vi "Evaluate Population Fitness.vi"(8 "error in":errorcluster, 11 "IPopulation in":refnum<class "IPopulation.lvclass">) -> (0 "error out":errorcluster, 3 "IPopulation out":refnum<class "IPopulation.lvclass">)   [LabVIEW 2016, in "IPopulation.lvclass"]
uses:
  IPopulation.lvclass
  IPopulation.lvclass/IPopulation.ctl
  IChromosome/IChromosome.lvclass
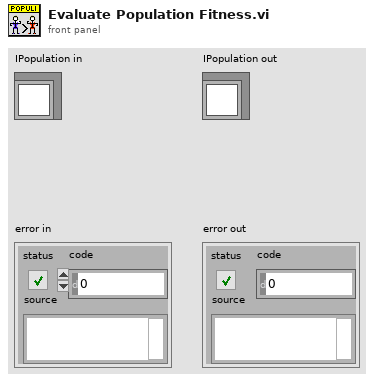
[diagram p1: front panel]
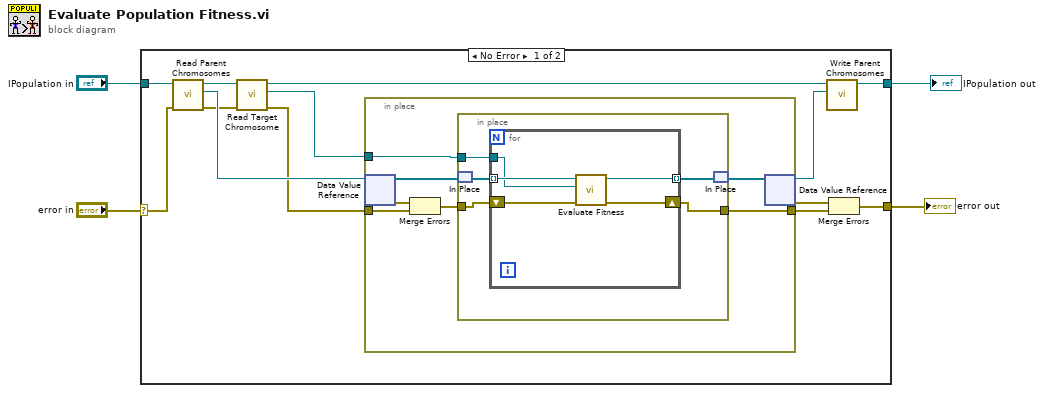
[diagram p0: block diagram]
diagram:
  n1 = case shown="No Error" "error in" {
    selector: "error in" -> [w7 w35]
    tunnel: [w17 w36] -> w4
    tunnel: "IPopulation in" -> [w14 w36]
    tunnel: [w11 w35] -> w1
    frame No Error {
      n2 = call "Read Parent Chromosomes.vi"("error in (no error)"=w7, "IPopulation in"=w14) -> ("error out"=w6:errorcluster, "Chromosomes"=w15:refnum<data-value>, "IPopulation out"=w10:refnum<class "IPopulation.lvclass">)  [unwired: 7 in]
      n3 = call "Read Target Chromosome.vi"("error in (no error)"=w6, "IPopulation in"=w10) -> ("error out"=w5:errorcluster, "IChromosome.lvclass"=w8:refnum<class "IChromosome.lvclass">, "IPopulation out"=w9:refnum<class "IPopulation.lvclass">)  [unwired: 7 in]
      n4 = in-place {
        in-place-border: [w24] -> w12
        in-place-border: w5 -> [w19]
        in-place-border: w8 -> [w18]
        n5 = in-place-dvr #1(w15) -> (w22:refnum<class "IChromosome.lvclass">[], w21:errorcluster)
        n6 = Merge Errors(w21, w19) -> (w20:errorcluster)
        n7 = in-place {
          in-place-border: w20 -> [w29]
          in-place-border: [w28] -> w24
          in-place-border: w18 -> [w25]
          n8 = in-place-match #2(w22) -> (w26:refnum<class "IChromosome.lvclass">[])
          n9 = for {
            tunnel: w26 -> [w31] mode=indexing
            shift-right: [w32] -> w28
            shift-left: w29 -> [w34]
            tunnel: [w33] -> w27 mode=indexing
            tunnel: w25 -> [w30]
            n10 = call "Evaluate Fitness.vi"("error in"=w34, "IChromosome Target in"=w30, "IChromosome in"=w31) -> ("error out"=w32:errorcluster, "IChromosome out"=w33:refnum<class "IChromosome.lvclass">)  [unwired: 7 in]
          }
          n11 = in-place-match #2(w27) -> (w23:refnum<class "IChromosome.lvclass">[])
        }
        n12 = in-place-dvr #1(w23) -> (w16:refnum<data-value>, w13:errorcluster)
      }
      n13 = call "Write Parent Chromosomes.vi"("Chromosomes"=w16, "IPopulation in"=w9) -> ("IPopulation out"=w17:refnum<class "IPopulation.lvclass">)  [unwired: 8 in, 1 out]
      n14 = Merge Errors(w13, w12) -> (w11:errorcluster)
    }
    frame Error {
    }
  }
  "error out" <- w1
  "IPopulation out" <- w4
